vi "UsrProfiles-Reinitialise.vi"(8 "error in":errorcluster) -> (0 "error out":errorcluster)   [LabVIEW 2020]
uses:
  Globals/gl_UsrProfiles globals.vi
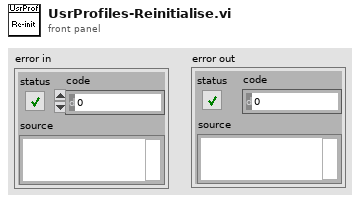
[diagram p1: front panel]
types:
  T1 = enum16{"Obtain queue", "Call window", "Call & send signal", "Release queue"}
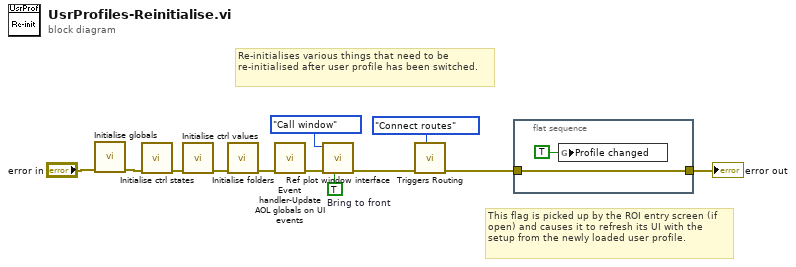
[diagram p0: block diagram]
diagram:
  w8 = TRUE  # Bring to front
  # "This flag is picked up by the ROI entry screen (if open) and causes it to refresh its UI with the setup from the newly loaded user profile."
  # "Re-initialises various things that need to be re-initialised after user profile has been switched."
  n1 = call "Initialise globals.vi"("error in (no error)"="error in") -> ("error out"=w11:errorcluster)  [unwired: 10 in]
  n2 = call "Initialise ctrl states.vi"("error in (no error)"=w11) -> ("error out"=w7:errorcluster)  [unwired: 10 in]
  n3 = call "Initialise ctrl values.vi"("error in (no error)"=w7) -> ("error out"=w6:errorcluster)  [unwired: 10 in]
  n4 = call "Initialise folders.vi"("error in (no error)"=w6) -> ("error out"=w5:errorcluster)  [unwired: 10 in]
  n5 = call "Event handler-Update AOL globals on UI events.vi"("error in (no error)"=w5) -> ("error out"=w4:errorcluster)  [unwired: 10 in]
  n6 = call "Ref plot window interface.vi"("Bring to front (F)"=w8, "error in (no error)"=w4, "Function"=T1."Call window") -> ("error out"=w9:errorcluster)  [unwired: 7 in, 1 out]
  n7 = call "Triggers Routing.vi"("Function"=enum16{"Connect routes", "Disconnect routes"}."Connect routes", "error in (no error)"=w9) -> ("error out (no error)"=w2:errorcluster)  [unwired: 9 in]
  n8 = flat-sequence {
    tunnel: w2 -> [w13]
    tunnel: [w13] -> w1
    frame #0 {
      n9 = global write "gl_UsrProfiles globals.vi" "Profile changed"(TRUE ("Profile changed")) -> ()
    }
  }
  "error out" <- w1
